vi "SQL_users_select.vi"() -> (2 "error out":errorcluster, 3 "用户信息":string[][](table))   [LabVIEW 2014]
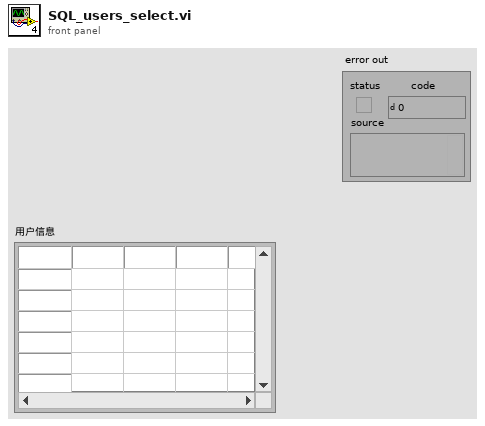
[diagram p1: front panel]
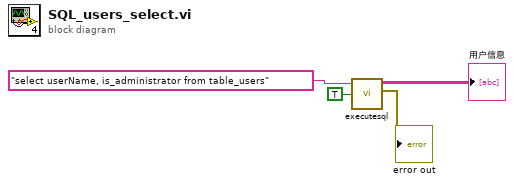
[diagram p0: block diagram]
diagram:
  n1 = call "executesql.vi"("Return Data (T)"=TRUE, "Command Text"="select userName, is_administrator from table_users") -> ("error out"=→"error out":errorcluster, "Data"=→"用户信息":string[][])  [unwired: 5 in]
